vi "SAC-Build Matfile Path.vi"(0 "State":T1) -> (4 "path":path, 8 "filestem":string)   [LabVIEW 2020]
uses:
  Typedefs/SAC-State.ctl
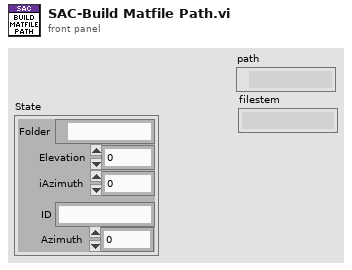
[diagram p1: front panel]
types:
  T1 = typedef "SAC-State.ctl" = cluster{"Folder":path, "Elevation":dbl, "iAzimuth":i32, "ID":string, "Azimuth":dbl}
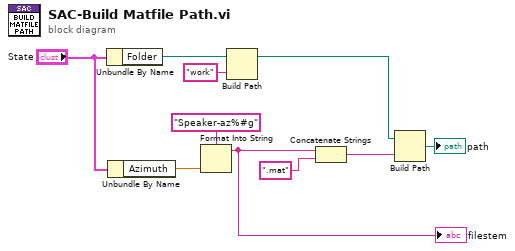
[diagram p0: block diagram]
diagram:
  n1 = Unbundle By Name("State") -> ("Folder"=w9:path)
  n2 = Unbundle By Name("State") -> ("Azimuth"=w8:dbl)
  n3 = Format Into String(format string="Speaker-az%#g", w8) -> (resulting string=w3:string)  [unwired: 2 in, 1 out]
  "filestem" <- w3
  n4 = Build Path(base path=w9, name or relative path="work") -> (appended path=w5:path)
  n5 = Concatenate Strings(w3, ".mat" ("format string")) -> (w1:string)
  n6 = Build Path(base path=w5, name or relative path=w1) -> (appended path=→"path":path)
